vi "Get Displacement from Steps_SubVI.vi"(6 "Step Indices":i32[](array[numeric]), 8 "Stride Length":dbl, 9 "North Displacement In":dbl, 10 "East Displacement In":dbl, 11 "Queue Elements In":T1[](array[typedef])) -> (2 "North Displacement Out":dbl, 3 "East Displacement Out":dbl, 5 "element":dbl)   [LabVIEW 2021]
uses:
  ProducerConsumer Data Cluster_TDef.ctl
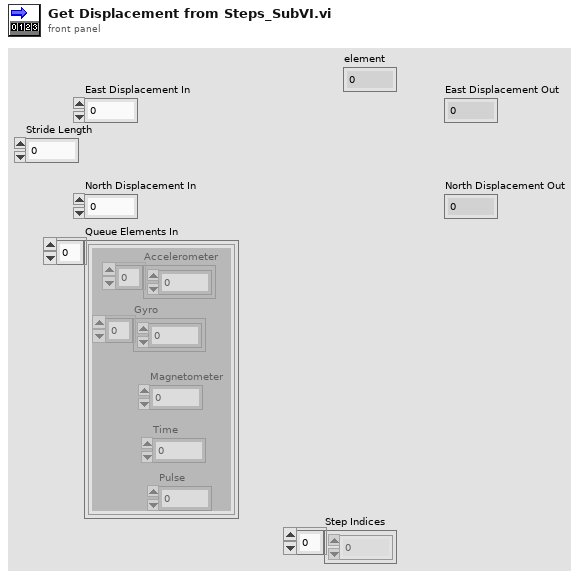
[diagram p1: front panel]
types:
  T1 = typedef "ProducerConsumer Data Cluster_TDef.ctl" = cluster{"Accelerometer":dbl[], "Gyro":dbl[], "Magnetometer":dbl, "Time":i32, "Pulse":dbl}
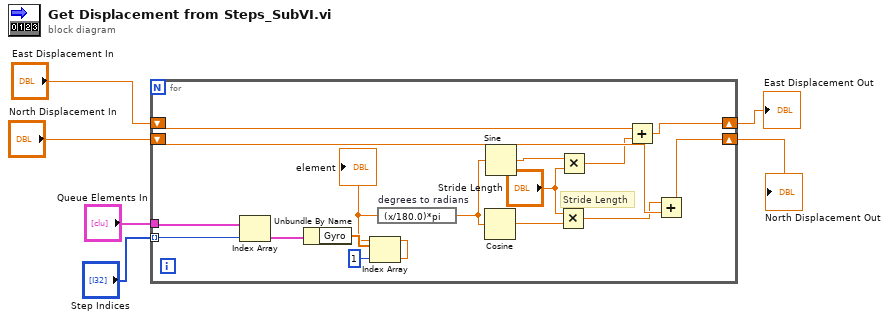
[diagram p0: block diagram]
diagram:
  n1 = for {
    tunnel: "Queue Elements In" -> [w22]
    shift-right: [w18] -> w4
    shift-left: "East Displacement In" -> [w17]
    shift-right: [w19] -> w5
    shift-left: "North Displacement In" -> [w20]
    tunnel: "Step Indices" -> [w12] mode=indexing
    # "Stride Length"
    n2 = Index Array(array=w22, index=w12) -> (element=w21:T1)
    n3 = Unbundle By Name(w21) -> ("Gyro"=w10:dbl[])
    n4 = Index Array(array=w10, index=1) -> (element=w8:dbl)
    "element" <- w8
    n5 = expression code="(x/180.0)*pi" "degrees to radians"(w8) -> (w7:dbl)
    n6 = Cosine(x=w7) -> (cos(x)=w14:dbl)
    n7 = Sine(x=w7) -> (sin(x)=w16:dbl)
    n8 = Multiply(x="Stride Length", y=w14) -> (x*y=w15:dbl)
    n9 = Multiply(x=w16, y="Stride Length") -> (x*y=w13:dbl)
    n10 = Add(x=w17, y=w13) -> (x+y=w18:dbl)
    n11 = Add(x=w15, y=w20) -> (x+y=w19:dbl)
  }
  "North Displacement Out" <- w5
  "East Displacement Out" <- w4
